vi "Draw Grid.vi"(7 "draw options":T2={"Background Color"=16777215, "Grid Color"=13816530, "Angle Units"=enum."Radians", "Draw Solid Background"=TRUE, "Draw Grid"=TRUE, "Grid Spacing"=1.0, "AutoScale"=TRUE, "Fit to Radius"=1.0, "data row options"=[]}, 9 "scaling info":T1={"pixels per unit"=1.0, "fit radius (units)"=1.0, "center point (pixels)"={"x"=0, "y"=0}}, 11 "picture in":picture) -> (3 "picture out":picture)   [LabVIEW 2017, in "NI_Robotics_2D Rangefinder Picture.lvlib"]
uses:
  <vilib>/robotics/Controls/2D Rangefinder/2D Rangefinder Picture/NI_Robotics_2D Rangefinder Picture.lvlib
  <vilib>/robotics/Controls/2D Rangefinder/2D Rangefinder Picture/Draw Options.ctl
  <vilib>/robotics/Controls/Utilities/Angle Units.ctl
  <vilib>/robotics/Controls/2D Rangefinder/2D Rangefinder Picture/Data Row Options.ctl
  <vilib>/robotics/Controls/2D Rangefinder/2D Rangefinder Picture/Scaling Info.ctl
  <vilib>/robotics/Controls/Utilities/NI_Robotics_Control Utilities.lvlib
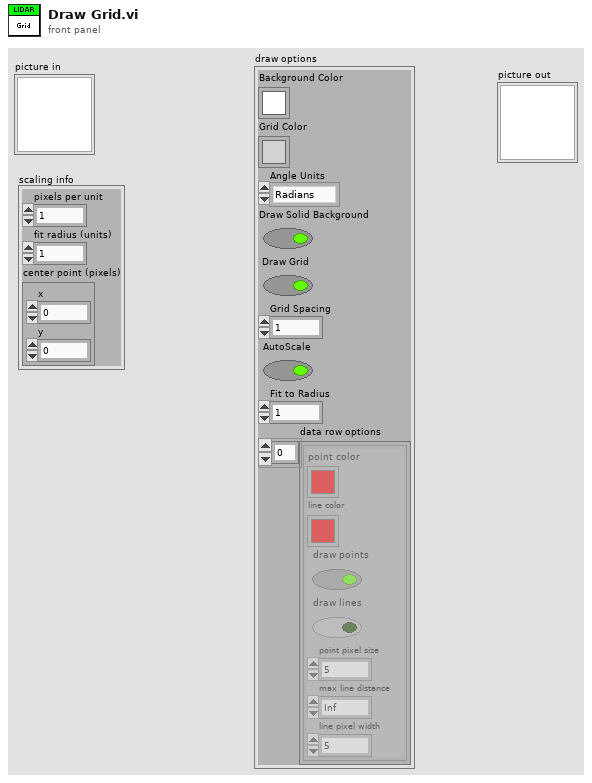
[diagram p1: front panel]
types:
  T1 = typedef "NI_Robotics_2D Rangefinder Picture.lvlib/Scaling Info.ctl" = cluster{"pixels per unit":dbl, "fit radius (units)":dbl, "center point (pixels)":cluster{"x":i16, "y":i16}}
  T2 = typedef "NI_Robotics_2D Rangefinder Picture.lvlib/Draw Options.ctl" = cluster{"Background Color":u32, "Grid Color":u32, "Angle Units":T3, "Draw Solid Background":bool, "Draw Grid":bool, "Grid Spacing":dbl, "AutoScale":bool, "Fit to Radius":dbl, "data row options":T4[]}
  T3 = typedef "NI_Robotics_Control Utilities.lvlib/Angle Units.ctl" = enum16{"Radians", "Degrees"}
  T4 = typedef "NI_Robotics_2D Rangefinder Picture.lvlib/Data Row Options.ctl" = cluster{"point color":u32, "line color":u32, "draw points":bool, "draw lines":bool, "point pixel size":u16, "max line distance":dbl, "line pixel width":u16}
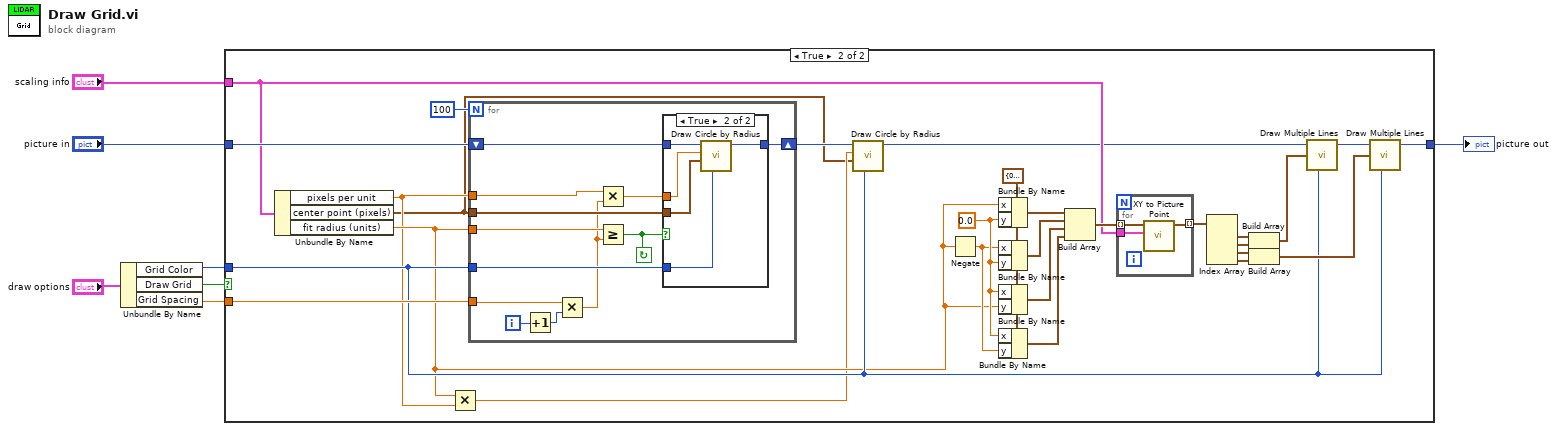
[diagram p0: block diagram]
diagram:
  n1 = Unbundle By Name("draw options") -> ("Grid Color"=w2:u32, "Draw Grid"=w6:bool, "Grid Spacing"=w1:dbl)
  n2 = case shown="True" w6 {
    tunnel: "picture in" -> [w8 w35]
    tunnel: [w8 w24] -> w4
    tunnel: "scaling info" -> [_ w26]
    tunnel: w2 -> [_ w13]
    tunnel: w1 -> [_ w36]
    frame False {
    }
    frame True {
      w33 = 0.0 ("y")
      w34 = cluster{"x":dbl, "y":dbl} {"x"=0.0, "y"=0.0} ("xy point (units)")
      n3 = Unbundle By Name(w26) -> ("pixels per unit"=w11:dbl, "center point (pixels)"=w9:cluster{"x":i16, "y":i16}, "fit radius (units)"=w12:dbl)
      n4 = Multiply(x=w12, y=w11) -> (x*y=w10:dbl)
      n5 = for {
        N: 100 -> [_]
        tunnel: w36 -> [w46]
        tunnel: w13 -> [w39]
        shift-right: [w43] -> w15
        shift-left: w35 -> [w44]
        tunnel: w12 -> [w45]
        tunnel: w9 -> [w42]
        tunnel: w11 -> [w41]
        i -> [w48]
        stop <- w37 continue-if-true
        n6 = Increment(x=w48) -> (x+1=w47:i32)
        n7 = Multiply(x=w46, y=w47) -> (x*y=w38:dbl)
        n8 = Multiply(x=w41, y=w38) -> (x*y=w40:dbl)
        n9 = Greater Or Equal?(x=w45, y=w38) -> (x >= y?=w37:bool)
        n10 = case shown="True" w37 {
          tunnel: w44 -> [w49 w54]
          tunnel: [w49 w53] -> w43
          tunnel: w42 -> [_ w52]
          tunnel: w40 -> [_ w51]
          tunnel: w39 -> [_ w50]
          frame False {
          }
          frame True {
            n11 = call <vilib>:"Draw Circle by Radius.vi"("color(black)"=w50, "pixel center"=w52, "radius"=w51, "picture"=w54) -> ("new picture"=w53:picture)  [unwired: 7 in]
          }
        }
      }
      n12 = call <vilib>:"Draw Circle by Radius.vi"("color(black)"=w13, "pixel center"=w9, "radius"=w10, "picture"=w15) -> ("new picture"=w14:picture)  [unwired: 7 in]
      n13 = Negate(x=w12) -> (-x=w32:dbl)
      n14 = Bundle By Name(cluster=w34, "x"=w12, "y"=w33) -> (w31:cluster{"x":dbl, "y":dbl})
      n15 = Bundle By Name(cluster=w34, "x"=w32, "y"=w33) -> (w30:cluster{"x":dbl, "y":dbl})
      n16 = Bundle By Name(cluster=w34, "x"=w33, "y"=w12) -> (w29:cluster{"x":dbl, "y":dbl})
      n17 = Bundle By Name(cluster=w34, "x"=w33, "y"=w32) -> (w28:cluster{"x":dbl, "y":dbl})
      n18 = Build Array(w31, w30, w29, w28) -> (w27:cluster{"x":dbl, "y":dbl}[])
      n19 = for {
        tunnel: w27 -> [w57] mode=indexing
        tunnel: w26 -> [w56]
        tunnel: [w55] -> w23 mode=indexing
        n20 = call <vilib>:"XY to Picture Point.vi"("scaling info"=w56, "xy point (units)"=w57) -> ("xy point (pixels)"=w55:cluster{"x":i16, "y":i16})  [unwired: 9 in]
      }
      n21 = Index Array(array=w23) -> (element #1=w22:cluster{"x":i16, "y":i16}, element #2=w21:cluster{"x":i16, "y":i16}, element #3=w20:cluster{"x":i16, "y":i16}, element #4=w19:cluster{"x":i16, "y":i16})  [unwired: 4 in]
      n22 = Build Array(w22, w21) -> (w18:cluster{"x":i16, "y":i16}[])
      n23 = Build Array(w20, w19) -> (w17:cluster{"x":i16, "y":i16}[])
      n24 = call <vilib>:"Draw Multiple Lines.vi"("picture"=w14, "line endpoints"=w18, "color(black)"=w13) -> ("new picture"=w25:picture)  [unwired: 6 in]
      n25 = call <vilib>:"Draw Multiple Lines.vi"("picture"=w25, "line endpoints"=w17, "color(black)"=w13) -> ("new picture"=w24:picture)  [unwired: 6 in]
    }
  }
  "picture out" <- w4
